vi "TCPListenJSON.vi"(8 "error in (no error)":errorcluster) -> (0 "error out":errorcluster, 3 "listener ID":refnum<k5>)   [LabVIEW 2013]
doc: "Sets up a TCP listener at a dynamically assigned port with service name \"SetList/JSON\". This is intended to designate the port used to send feedback requests to SetList."
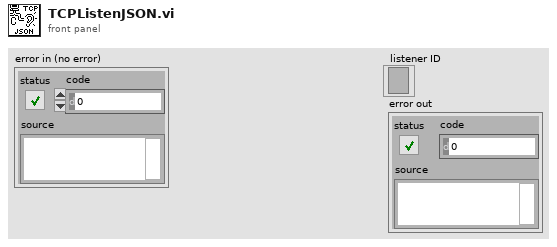
[diagram p1: front panel]
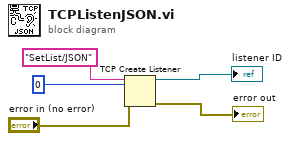
[diagram p0: block diagram]
diagram:
  n1 = TCP Create Listener(8:"error in (no error)", 10:u16 0 ("port"), 11:"SetList/JSON" ("service name")) -> (0:→"error out":errorcluster, 3:→"listener ID":refnum<k5>)  [unwired: 2 in, 1 out]
